vi "niRFUtil CONV DBL to I32.vi"(7 "Numeric (DBL)":dbl format="%#.12g") -> (8 "Numeric (I32)":i32)   [LabVIEW 2016, in "niRFUtil.lvlib"]
uses:
  niRFUtil.lvlib
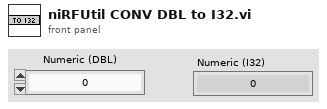
[diagram p1: front panel]
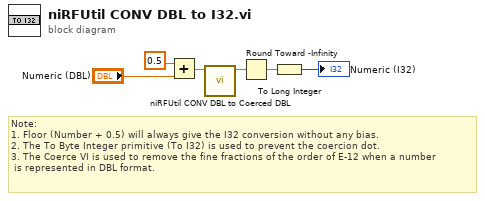
[diagram p0: block diagram]
diagram:
  # "Note:\n1. Floor (Number + 0.5) will always give the I32 conversion without any bias.\n2. The To Byte Integer primitive (To I32) is used to prevent the coercion dot.\n3. The Coerce VI is used to remove the fine fractions of the order of E-12 when a number\n is represented in DBL format."
  n1 = Add(x=0.5, y="Numeric (DBL)") -> (x+y=w4:dbl)
  n2 = call "niRFUtil CONV DBL to Coerced DBL.vi"("Numeric In (DBL)"=w4) -> ("Coerced Numeric Out (DBL)"=w3:dbl)  [unwired: 10 in]
  n3 = Round Toward -Infinity(1:w3) -> (0:w6:dbl)
  n4 = To Long Integer(number=w6) -> (32bit integer=→"Numeric (I32)":i32)
